vi "Wysylanie UDP do SbRIO.vi"(7 "Cluster":T2, 10 "output cluster":T1) -> (1 "error out udp":errorcluster, 2 "output cluster 2":T1, 3 "connection ID out":refnum<k16>, 4 "stop error ?":bool)   [LabVIEW 2015]
uses:
  QMH Fundamentals - Message Cluster.ctl
panel:
  out "length":i32
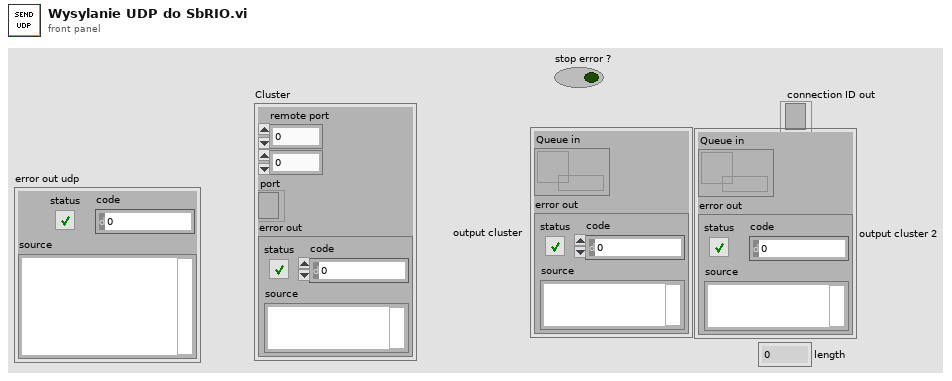
[diagram p1: front panel]
types:
  T1 = cluster{"Queue in":refnum<queue>, "error out":errorcluster}
  T2 = cluster{"remote port":u16, u32, "port":refnum<k16>, "error out":errorcluster}
  T3 = typedef "QMH Fundamentals - Message Cluster.ctl" = cluster{"Message":string, "Message Data":variant}
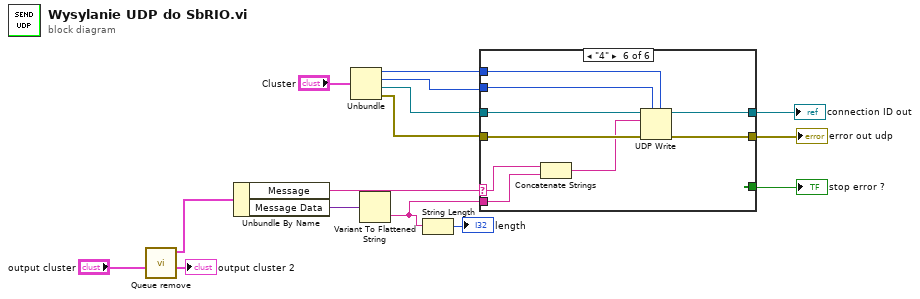
[diagram p0: block diagram]
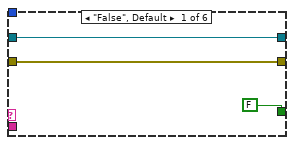
[diagram p2: hidden frame]
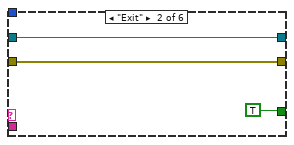
[diagram p3: hidden frame]
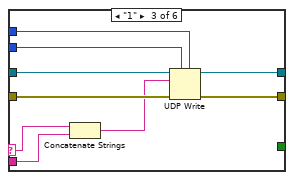
[diagram p4: hidden frame]
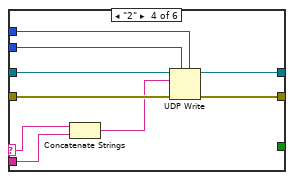
[diagram p5: hidden frame]
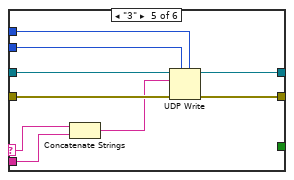
[diagram p6: hidden frame]
diagram:
  n1 = call "Queue remove.vi"("output cluster"="output cluster") -> ("output cluster 2"=→"output cluster 2":T1, "Message Cluster"=w3:T3)  [unwired: 9 in]
  n2 = Unbundle By Name(w3) -> ("Message"=w6:string, "Message Data"=w7:variant)
  n3 = Unbundle("Cluster") -> ("remote port"=w12:u16, w13:u32, "port"=w11:refnum<k16>, "error out"=w10:errorcluster)
  n4 = Variant To Flattened String(Variant=w7) -> (data string=w5:string)  [unwired: 1 out]
  n5 = String Length(string=w5) -> (length=→"length":i32)
  n6 = case shown="\"4\"" w6 {
    selector: w6 -> [_ _ w22 w31 w40 w49]
    tunnel: w13 -> [_ _ w26 w35 w44 w53]
    tunnel: w12 -> [_ _ w25 w34 w43 w52]
    tunnel: w11 -> [w16 w19 w27 w36 w45 w54]
    tunnel: w10 -> [w18 w21 w30 w39 w48 w57]
    tunnel: [w18 w21 w29 w38 w47 w56] -> w14
    tunnel: [FALSE TRUE _ _ _ _] -> w15
    tunnel: w5 -> [_ _ w23 w32 w41 w50]
    tunnel: [w16 w19 w28 w37 w46 w55] -> w8
    frame "False", Default {
    }
    frame "Exit" {
    }
    frame "1" {
      n7 = Concatenate Strings(w22, w23) -> (w24:string)
      n8 = UDP Write(address=w26, port or service name=w25, connection ID=w27, data in=w24, 8:w30) -> (error out=w29:errorcluster, 3:w28:refnum<k16>)  [unwired: 1 in]
    }
    frame "2" {
      n9 = Concatenate Strings(w31, w32) -> (w33:string)
      n10 = UDP Write(address=w35, port or service name=w34, connection ID=w36, data in=w33, 8:w39) -> (error out=w38:errorcluster, 3:w37:refnum<k16>)  [unwired: 1 in]
    }
    frame "3" {
      n11 = Concatenate Strings(w40, w41) -> (w42:string)
      n12 = UDP Write(address=w44, port or service name=w43, connection ID=w45, data in=w42, 8:w48) -> (error out=w47:errorcluster, 3:w46:refnum<k16>)  [unwired: 1 in]
    }
    frame "4" {
      n13 = Concatenate Strings(w49, w50) -> (w51:string)
      n14 = UDP Write(address=w53, port or service name=w52, connection ID=w54, data in=w51, 8:w57) -> (error out=w56:errorcluster, 3:w55:refnum<k16>)  [unwired: 1 in]
    }
  }
  "stop error ?" <- w15
  "error out udp" <- w14
  "connection ID out" <- w8
